vi "Configure LIN Trigger Source.vi"(0 "VISA resource name":refnum<visa-resource-name>, 5 "Trigger Source (0: Channel 1)":u16(ring) items=["Channel 1", "Channel 2", "Channel 3", "Channel 4", "DIG 0", "DIG 1", "DIG 2", "DIG 3", "DIG 4", "DIG 5", "DIG 6", "DIG 7", "DIG 8", "DIG 9", "DIG 10", "DIG 11", "DIG 12", "DIG 13", "DIG 14", "DIG 15", "EXT"], 7 "Signal (1: Rx)":u16(ring)=1 items=["LIN", "RX", "TX"], 9 "Baud Rate (0: 2400)":u16(ring) items=["2400", "9600", "19200"], 11 "error in (no error)":errorcluster) -> (4 "VISA resource name out":refnum<visa-resource-name>, 15 "error out":errorcluster)   [LabVIEW 2017, in "Agilent 6000 Series.lvlib"]
doc: "This VI configures the LIN (Local Interconnect Network) trigger. \n\n<B>NOTE:</B>\n\nThis VI is only valid for 6000 Series models. An error will be thrown if this VI is run with 5000 Series scopes."
uses:
  <instrlib>/Agilent 6000 Series/Agilent 6000 Series.lvlib
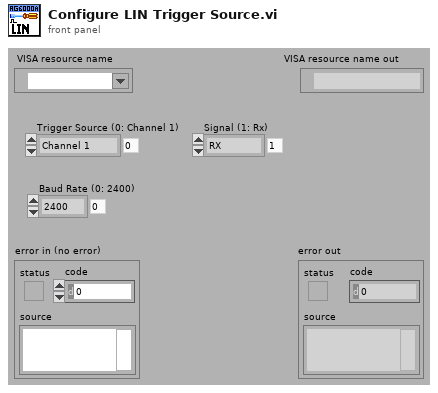
[diagram p1: front panel]
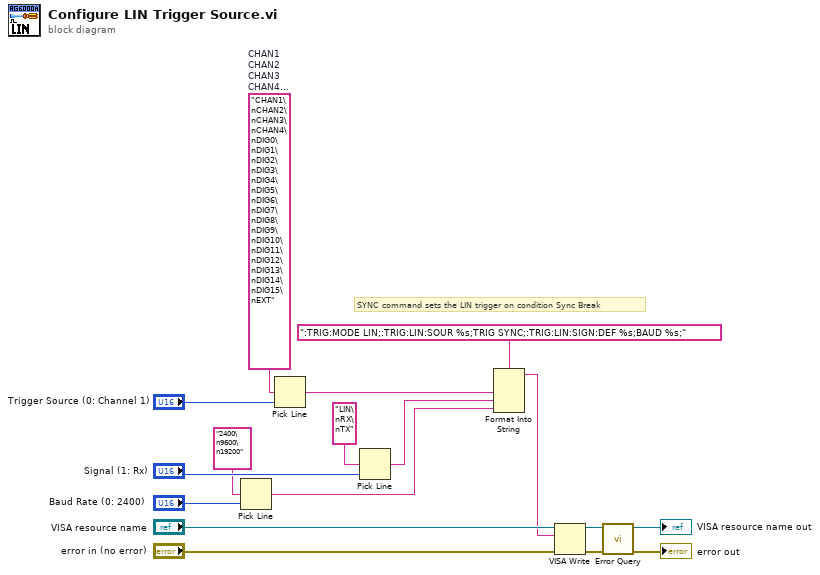
[diagram p0: block diagram]
diagram:
  w10 = "CHAN1\nCHAN2\nCHAN3\nCHAN4\nDIG0\nDIG1\nDIG2\nDIG3\nDIG4\nDIG5\nDIG6\nDIG7\nDIG8\nDIG9\nDIG10\nDIG11\nDIG12\nDIG13\nDIG14\nDIG15\nEXT"  # CHAN1 CHAN2 CHAN3 CHAN4 DIG0 DIG1 DIG2 DIG3 DIG4 DIG5 DIG6 DIG7 DIG8 DIG9 DIG10 DIG11 DIG12 DIG13 DIG14 DIG15 EXT
  # "SYNC command sets the LIN trigger on condition Sync Break"
  n1 = Pick Line(multi-line string="2400\n9600\n19200", line index="Baud Rate (0: 2400)") -> (output string=w2:string)  [unwired: 1 in]
  n2 = Pick Line(multi-line string=w10, line index="Trigger Source (0: Channel 1)") -> (output string=w4:string)  [unwired: 1 in]
  n3 = Pick Line(multi-line string="LIN\nRX\nTX", line index="Signal (1: Rx)") -> (output string=w3:string)  [unwired: 1 in]
  n4 = Format Into String(format string=":TRIG:MODE LIN;:TRIG:LIN:SOUR %s;TRIG SYNC;:TRIG:LIN:SIGN:DEF %s;BAUD %s;" ("Source Command"), w4, w3, w2) -> (resulting string=w1:string)  [unwired: 2 in, 1 out]
  n5 = VISA Write(VISA resource name="VISA resource name", write buffer=w1, error in (no error)="error in (no error)") -> (VISA resource name out=w13:refnum<visa-resource-name>, error out=w12:errorcluster)  [unwired: 1 out]
  n6 = call <instrlib>:"Error Query.vi"("error in (no error)"=w12, "VISA resource name"=w13) -> ("error out"=→"error out":errorcluster, "VISA resource name out"=→"VISA resource name out":refnum<visa-resource-name>)  [unwired: 6 in, 2 out]
